vi "Feet to Codes.vi"(1 "Feet":dbl) -> (0 "Codes":dbl)   [LabVIEW 2012]
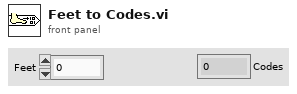
[diagram p1: front panel]
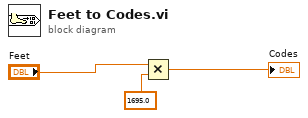
[diagram p0: block diagram]
diagram:
  n1 = Multiply(x="Feet", y=1695.0) -> (x*y=→"Codes":dbl)
